vi "Read MTi Theta Offset.vi"(8 "error in (no error)":errorcluster, 11 "Attitude Observer in":refnum<class "Attitude Observer.lvclass">) -> (0 "error out":errorcluster, 2 "MTi Theta Offset":dbl[](array[numeric])=[0.0, 0.0, 180.0], 3 "Attitude Observer out":refnum<class "Attitude Observer.lvclass">)   [LabVIEW 2014, in "Observer Library.lvlib" / "Attitude Observer.lvclass"]
uses:
  Attitude Observer.lvclass
  Attitude Observer.lvclass/Attitude Observer.ctl
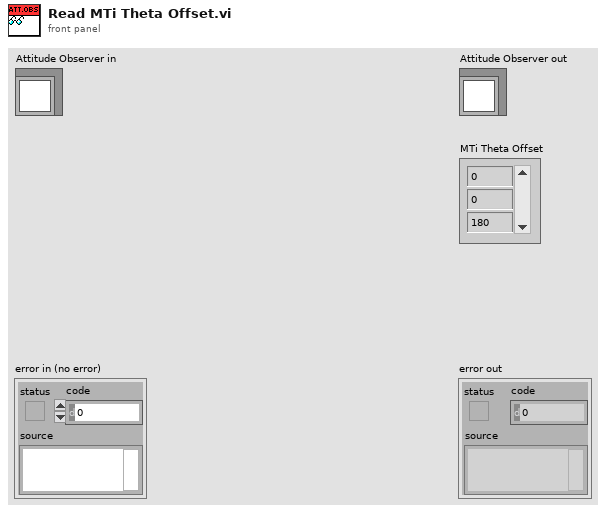
[diagram p1: front panel]
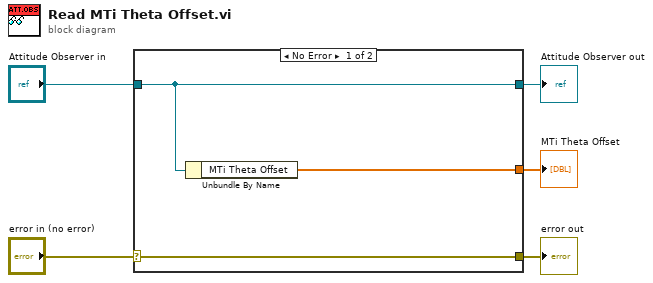
[diagram p0: block diagram]
diagram:
  n1 = case shown="No Error" "error in (no error)" {
    selector: "error in (no error)" -> [w8 w9]
    tunnel: [w8 w9] -> w4
    tunnel: [w7 w10] -> w2
    tunnel: "Attitude Observer in" -> [w7 w10]
    tunnel: [w6 _] -> w1
    frame No Error {
      n2 = Unbundle By Name(w7) -> ("MTi Theta Offset"=w6:dbl[])
    }
    frame Error {
    }
  }
  "error out" <- w4
  "Attitude Observer out" <- w2
  "MTi Theta Offset" <- w1
